vi "CMD_MOVECIR.vi"(6 "Gantry in":refnum<class "Gantry.lvclass">, 8 "error in (no error)":errorcluster, 10 "Arguments":string[](array[string]), 11 "gScript Interpreter in":refnum<class "gScript Interpreter.lvclass">) -> (0 "error out":errorcluster, 3 "gScript Interpreter out":refnum<class "gScript Interpreter.lvclass">, 4 "Gantry out":refnum<class "Gantry.lvclass">)   [LabVIEW 2024, in "gScript Interpreter.lvclass"]
uses:
  gScript Interpreter.lvclass
  Shared Components/Gantry Class/Gantry.lvclass
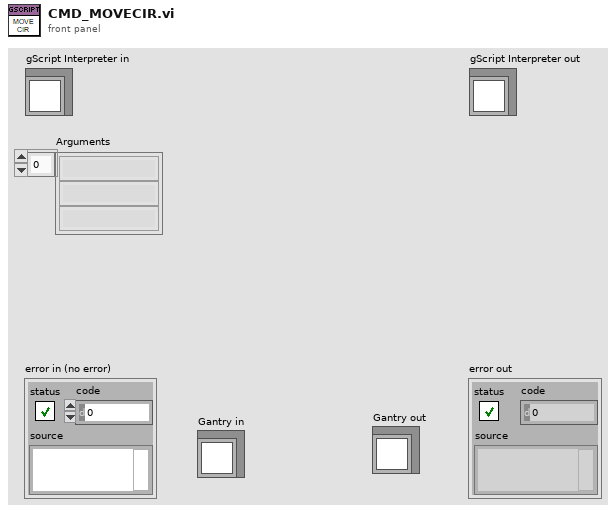
[diagram p1: front panel]
types:
  T1 = typedef "Memory Cell.ctl" = cluster{"type":T2, "x":dbl, "y":dbl, "z":dbl, "w":dbl}
  T2 = typedef "Memory Cell Type Enum.ctl" = enum16{"integer", "float", "vector", "rotation"}
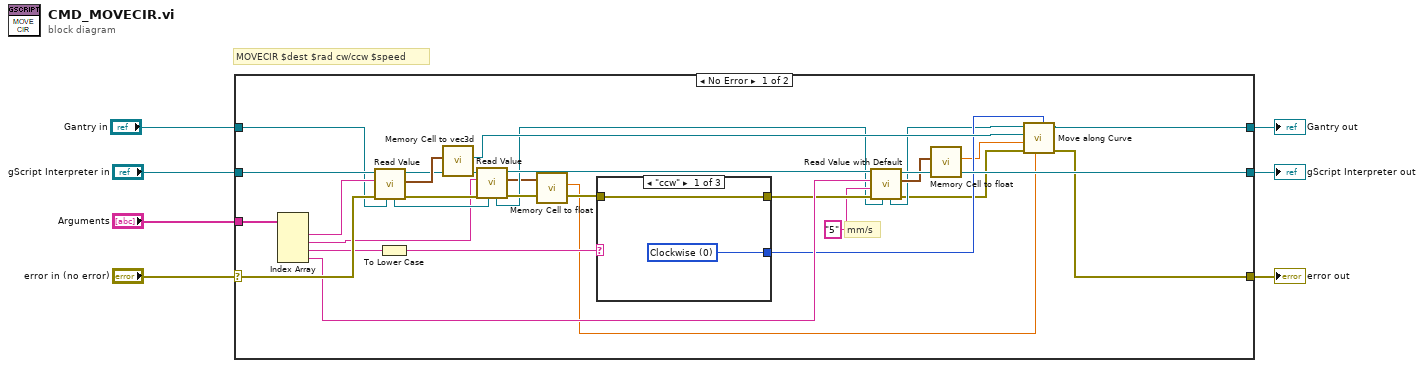
[diagram p0: block diagram]
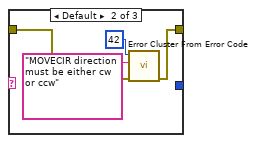
[diagram p2: hidden frame]
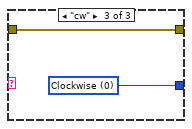
[diagram p3: hidden frame]
diagram:
  # "MOVECIR $dest $rad cw/ccw $speed"
  n1 = case shown="No Error" "error in (no error)" {
    selector: "error in (no error)" -> [w34 w47]
    tunnel: [w8 w47] -> w6
    tunnel: [w29 w46] -> w4
    tunnel: "gScript Interpreter in" -> [w35 w46]
    tunnel: "Arguments" -> [w33 _]
    tunnel: "Gantry in" -> [w28 w45]
    tunnel: [w36 w45] -> w1
    frame No Error {
      # "mm/s"
      n2 = Index Array(array=w33) -> (element #1=w32:string, element #2=w11:string, element #3=w26:string, element #4=w27:string)  [unwired: 4 in]
      n3 = call-dynamic "Read Value.vi"("Gantry in"=w28, "error in (no error)"=w34, "String in"=w32, "gScript Interpreter in"=w35) -> ("error out"=w15:errorcluster, "Memory Cell"=w31:T1, "gScript Interpreter out"=w17:refnum<class "gScript Interpreter.lvclass">, "Gantry out"=w13:refnum<class "Gantry.lvclass">)  [unwired: 4 in]
      n4 = To Lower Case(string=w26) -> (all lower case string=w25:string)
      n5 = call "Memory Cell to vec3d.vi"("Memory Cell"=w31) -> ("Vec3d out"=w30:refnum<class "Vec3d.lvclass">)  [unwired: 10 in]
      n6 = call-dynamic "Read Value.vi"("Gantry in"=w13, "error in (no error)"=w15, "String in"=w11, "gScript Interpreter in"=w17) -> ("error out"=w14:errorcluster, "Memory Cell"=w9:T1, "gScript Interpreter out"=w16:refnum<class "gScript Interpreter.lvclass">, "Gantry out"=w12:refnum<class "Gantry.lvclass">)  [unwired: 4 in]
      n7 = call "Memory Cell to float.vi"("Memory Cell"=w9) -> ("float out"=w10:dbl)  [unwired: 10 in]
      n8 = case shown="\"ccw\"" w25 {
        tunnel: w14 -> [w37 w42 w44]
        tunnel: [w37 w41 w44] -> w23
        tunnel: [w38 _ w43] -> w24
        frame "ccw" {
          w38 = u16 0 items=["Clockwise", "Counter-clockwise"] ("direction")
        }
        frame Default {
          n9 = call <vilib>:"Error Cluster From Error Code.vi"("error in (no error)"=w42, "error message (\"\")"="MOVECIR direction must be either cw or ccw" ("error message (\"\")"), "error code (0)"=42) -> ("error out"=w41:errorcluster)  [unwired: 6 in]
        }
        frame "cw" {
          w43 = u16 0 items=["Clockwise", "Counter-clockwise"] ("direction")
        }
      }
      n10 = call "Read Value with Default.vi"("Gantry in"=w12, "error in (no error)"=w23, "Default"="5", "String in"=w27, "gScript Interpreter in"=w16) -> ("error out"=w20:errorcluster, "Memory Cell"=w22:T1, "gScript Interpreter out"=w29:refnum<class "gScript Interpreter.lvclass">, "Gantry out"=w21:refnum<class "Gantry.lvclass">)  [unwired: 3 in]
      n11 = call "Memory Cell to float.vi"("Memory Cell"=w22) -> ("float out"=w19:dbl)  [unwired: 10 in]
      n12 = call-dynamic "Move along Curve.vi"("direction"=w24, "Radius"=w10, "error in"=w20, "Speed"=w19, "Destination"=w30, "Gantry in"=w21) -> ("error out"=w8:errorcluster, "Gantry out"=w36:refnum<class "Gantry.lvclass">)  [unwired: 4 in]
    }
    frame Error {
    }
  }
  "error out" <- w6
  "gScript Interpreter out" <- w4
  "Gantry out" <- w1
